vi "_Buffer_To_AllElements.vi"(10 "count (-1: all)":i32=-1, 11 "Buffer":refnum<class "VariantBuffer.lvclass">) -> (3 "elements":variant[](array[variant]))   [LabVIEW 2013, in "CircularBuffer.lvlib" / "VariantBuffer.lvclass"]
uses:
  VariantBuffer.lvclass
  VariantBuffer.lvclass/VariantBuffer.ctl
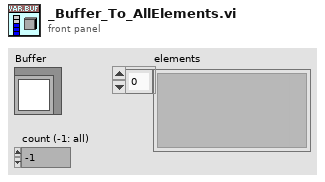
[diagram p1: front panel]
types:
  T1 = typedef "CircularBuffer.lvlib/VariantBuffer.lvclass/buffer-type -- enum.ctl" = enum16{"Queue", "Stack"}
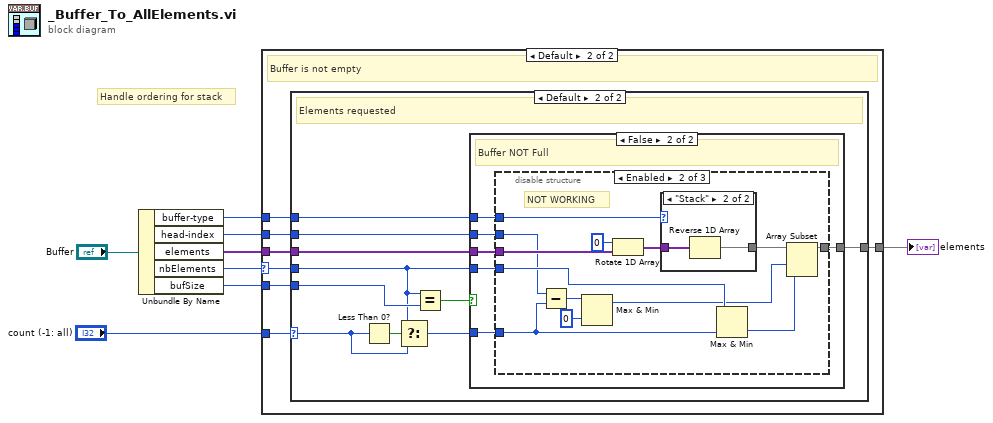
[diagram p0: block diagram]
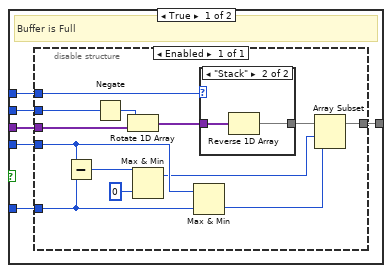
[diagram p4: hidden frame]
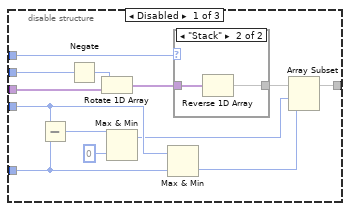
[diagram p6: hidden frame]
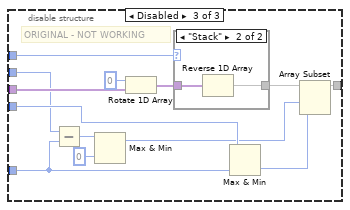
[diagram p9: hidden frame]
diagram:
  # "Handle ordering for stack"
  n1 = Unbundle By Name("Buffer") -> ("buffer-type"=w1:T1, "head-index"=w8:i32, "elements"=w5:variant[], "nbElements"=w3:i32, "bufSize"=w4:i32)
  n2 = case shown="Default" w3 {
    selector: w3 -> [_ w11]
    tunnel: "count (-1: all)" -> [_ w10]
    tunnel: w8 -> [_ w15]
    tunnel: [_ w14] -> w7
    tunnel: w5 -> [_ w13]
    tunnel: w4 -> [_ w12]
    tunnel: w1 -> [_ w9]
    frame 0 {
      # "Buffer is empty"
    }
    frame Default {
      # "Buffer is not empty"
      n3 = case shown="Default" w10 {
        selector: w10 -> [_ w17]
        tunnel: w15 -> [_ w23]
        tunnel: [_ w22] -> w14
        tunnel: w13 -> [_ w21]
        tunnel: w12 -> [_ w19]
        tunnel: w11 -> [_ w18]
        tunnel: w9 -> [_ w16]
        frame 0 {
          # "No elements are requested"
        }
        frame Default {
          # "Elements requested"
          n4 = Less Than 0?(x=w17) -> (x < 0?=w24:bool)
          n5 = Select(t=w18, s=w24, f=w17) -> (s? t:f=w25:i32)
          n6 = Equal?(x=w18, y=w19) -> (x = y?=w20:bool)
          n7 = case shown="False" w20 {
            tunnel: w21 -> [w31 w53]
            tunnel: [w30 w52] -> w22
            tunnel: w25 -> [w29 w51]
            tunnel: w23 -> [w28 w50]
            tunnel: w18 -> [w27 w49]
            tunnel: w16 -> [w26 w48]
            frame True {
              # "Buffer is Full"
              n8 = disable-structure shown="Enabled" {
                disable-tunnel: w31 -> [w44]
                disable-tunnel: [w43] -> w30
                disable-tunnel: w29 -> [w39]
                disable-tunnel: w28 -> [w37]
                disable-tunnel: w27 -> [w36]
                disable-tunnel: w26 -> [w35]
                frame Enabled {
                  n9 = Subtract(x=w36, y=w39) -> (x-y=w41:i32)
                  n10 = Negate(x=w37) -> (-x=w42:i32)
                  n11 = Rotate 1D Array(1:w44, 2:w42) -> (0:w34:variant[])
                  n12 = Max & Min(x=w41, y=0) -> (max(x,y)=w32:i32)  [unwired: 1 out]
                  n13 = Max & Min(x=w36, y=w39) -> (min(x,y)=w38:i32)  [unwired: 1 out]
                  n14 = case shown="\"Stack\"" w35 {
                    tunnel: w34 -> [w45 w47]
                    tunnel: [w45 w46] -> w33
                    frame "Queue" {
                    }
                    frame "Stack" {
                      n15 = Reverse 1D Array(array=w47) -> (reversed array=w46:variant[])
                    }
                  }
                  n16 = Array Subset(array=w33, index=w32, length=w38) -> (w43:variant[])
                }
              }
            }
            frame False {
              # "Buffer NOT Full"
              n17 = disable-structure shown="Enabled" {
                disable-tunnel: w53 -> [w66 w75 w91]
                disable-tunnel: [w65 w79 w95] -> w52
                disable-tunnel: w51 -> [w61 w78 w94]
                disable-tunnel: w50 -> [w59 w71 w88]
                disable-tunnel: w49 -> [w58 w73 w89]
                disable-tunnel: w48 -> [w57 w76 w92]
                frame Disabled {
                  n18 = Subtract(x=w58, y=w61) -> (x-y=w63:i32)
                  n19 = Negate(x=w59) -> (-x=w64:i32)
                  n20 = Rotate 1D Array(1:w66, 2:w64) -> (0:w56:variant[])
                  n21 = Max & Min(x=w63, y=0) -> (max(x,y)=w54:i32)  [unwired: 1 out]
                  n22 = Max & Min(x=w58, y=w61) -> (min(x,y)=w60:i32)  [unwired: 1 out]
                  n23 = case shown="\"Stack\"" w57 {
                    tunnel: w56 -> [w67 w69]
                    tunnel: [w67 w68] -> w55
                    frame "Queue" {
                    }
                    frame "Stack" {
                      n24 = Reverse 1D Array(array=w69) -> (reversed array=w68:variant[])
                    }
                  }
                  n25 = Array Subset(array=w55, index=w54, length=w60) -> (w65:variant[])
                }
                frame Enabled {
                  # "NOT WORKING"
                  n26 = Subtract(x=w71, y=w78) -> (x-y=w81:i32)
                  n27 = Max & Min(x=w81, y=0) -> (max(x,y)=w70:i32)  [unwired: 1 out]
                  n28 = Rotate 1D Array(1:w75, 2:0 ("n")) -> (0:w77:variant[])
                  n29 = case shown="\"Stack\"" w76 {
                    tunnel: w77 -> [w83 w85]
                    tunnel: [w83 w84] -> w74
                    frame "Queue" {
                    }
                    frame "Stack" {
                      n30 = Reverse 1D Array(array=w85) -> (reversed array=w84:variant[])
                    }
                  }
                  n31 = Max & Min(x=w73, y=w78) -> (min(x,y)=w82:i32)  [unwired: 1 out]
                  n32 = Array Subset(array=w74, index=w70, length=w82) -> (w79:variant[])
                }
                frame Disabled {
                  # "ORIGINAL - NOT WORKING"
                  n33 = Subtract(x=w88, y=w94) -> (x-y=w97:i32)
                  n34 = Max & Min(x=w97, y=0) -> (max(x,y)=w86:i32)  [unwired: 1 out]
                  n35 = Rotate 1D Array(1:w91, 2:0 ("n")) -> (0:w93:variant[])
                  n36 = case shown="\"Stack\"" w92 {
                    tunnel: w93 -> [w99 w101]
                    tunnel: [w99 w100] -> w90
                    frame "Queue" {
                    }
                    frame "Stack" {
                      n37 = Reverse 1D Array(array=w101) -> (reversed array=w100:variant[])
                    }
                  }
                  n38 = Max & Min(x=w89, y=w94) -> (min(x,y)=w98:i32)  [unwired: 1 out]
                  n39 = Array Subset(array=w90, index=w86, length=w98) -> (w95:variant[])
                }
              }
            }
          }
        }
      }
    }
  }
  "elements" <- w7
